vi "Temperature Warnings.vi"() -> ()   [LabVIEW 2019]
doc: "本VI用于判定基于当前温度值和边界设置的字符串，该字符串输出至气象站。\n\n输入：当前温度值（双精度）、最低温度值（双精度）和最高温度值（双精度）。\n输出：警告文本（字符串）和警告？（布尔）。"
panel:
  out "气象数据输出":T1={"当前温度"=0.0, "最高温度"=0.0, "最低温度"=0.0, "警告文本"="无警告", "警告？"=FALSE}
  in  "气象数据输入":T1={"当前温度"=0.0, "最高温度"=0.0, "最低温度"=0.0, "警告文本"="无警告", "警告？"=FALSE}
  out "错误输出":cluster{"状态":bool, "代码":i32, "源":string}
  in  "错误输入":cluster{"状态":bool, "代码":i32, "源":string}
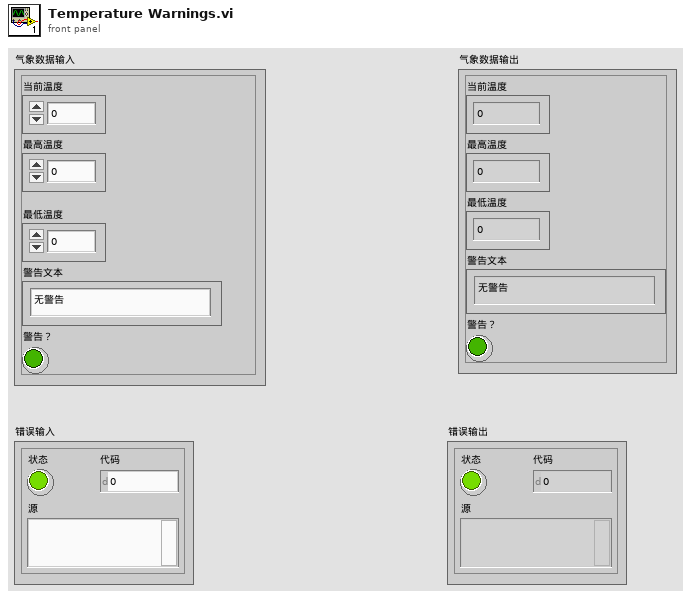
[diagram p1: front panel]
types:
  T1 = cluster{"当前温度":dbl, "最高温度":dbl, "最低温度":dbl, "警告文本":string, "警告？":bool}
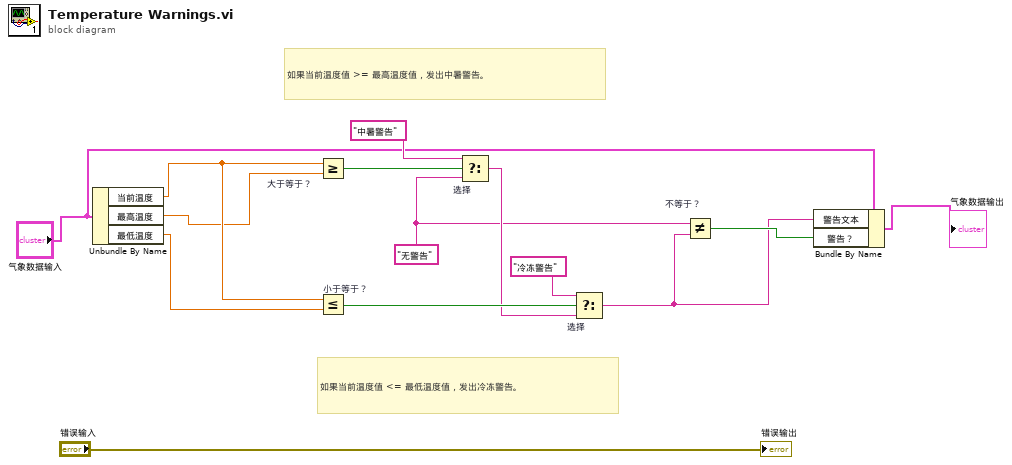
[diagram p0: block diagram]
diagram:
  w9 = "无警告" ("f")
  # "如果当前温度值 >= 最高温度值，发出中暑警告。"
  # "如果当前温度值 <= 最低温度值，发出冷冻警告。"
  n1 = Unbundle By Name("气象数据输入") -> ("当前温度"=w7:dbl, "最高温度"=w5:dbl, "最低温度"=w6:dbl)
  n2 = Greater Or Equal? "大于等于？"(x=w7, y=w5) -> (x >= y?=w14:bool)
  n3 = Less Or Equal? "小于等于？"(x=w7, y=w6) -> (x <= y?=w11:bool)
  n4 = Select "选择"(t="中暑警告", s=w14, f=w9) -> (s? t:f=w10:string)
  n5 = Select "选择"(t="冷冻警告", s=w11, f=w10) -> (s? t:f=w3:string)
  n6 = Not Equal? "不等于？"(x=w9, y=w3) -> (x != y?=w4:bool)
  n7 = Bundle By Name(cluster="气象数据输入", "警告文本"=w3, "警告？"=w4) -> (→"气象数据输出":T1)
  "错误输出" <- "错误输入"
